vi "User Plugin.vi"(5 "Initialize":bool, 8 "error in (no error)":errorcluster, 10 "ParamValues":sgl[](array[numeric]), 11 "DSI Reference":refnum<class "DCM-DSI-UserFuelExample.lvclass">) -> (0 "error out":errorcluster, 3 "DSI Reference":refnum<class "DCM-DSI-UserFuelExample.lvclass">, 4 "Results":T1[](array[typedef]), 6 "ParamNames":string[](array[string]))   [LabVIEW 2016, in "DCM-DSI-UserFuelExample.lvclass"]
uses:
  DCM-DSI-UserFuelExample.lvclass
  D:/PCG/Products/DCM/Software/DCM-DSI/Classes/DCM-DSI/DCM-DSI.lvclass
  DCM-DSI/UserParameter.ctl
  DCM-DSI/Channel.ctl
  DCM-DSI/Read Channels.vi
  DCM-DSI/Read EPTx Data.vi
  DCM-DSI/Read dt.vi
  DCM-DSI/Write Channels.vi
  DCM-DSI/DCM-DSI.lvclass
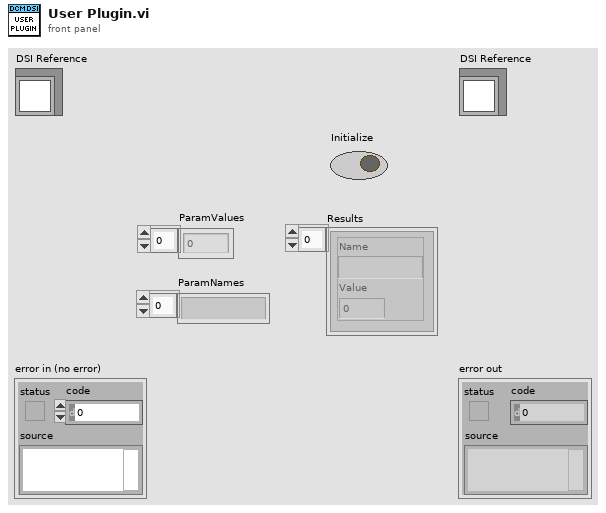
[diagram p1: front panel]
types:
  T1 = typedef "DCM-DSI.lvclass/UserParameter.ctl" = cluster{"Name":string, "Value":dbl}
  T2 = typedef "DCM-DSI.lvclass/Channel.ctl" = cluster{"Name":string, "Unit":string, "Value":sgl}
  T3 = cluster{"XArray":sgl[], "YArray":sgl[], "ZArray":dbl[][]}
  T4 = typedef "EPTx - RevA - RT.lvlib/EPTxData.ctl" = cluster{"Sync":bool, "CurrentCAD":sgl, "Speed [RPM]":sgl, "Config":bool, "Rcvg Primary":bool, "Stall":bool, "Overflow":bool, "Ratio Error":bool, "Pattern Error":bool, "Aux Warning":bool, "Watchdog Error":bool}
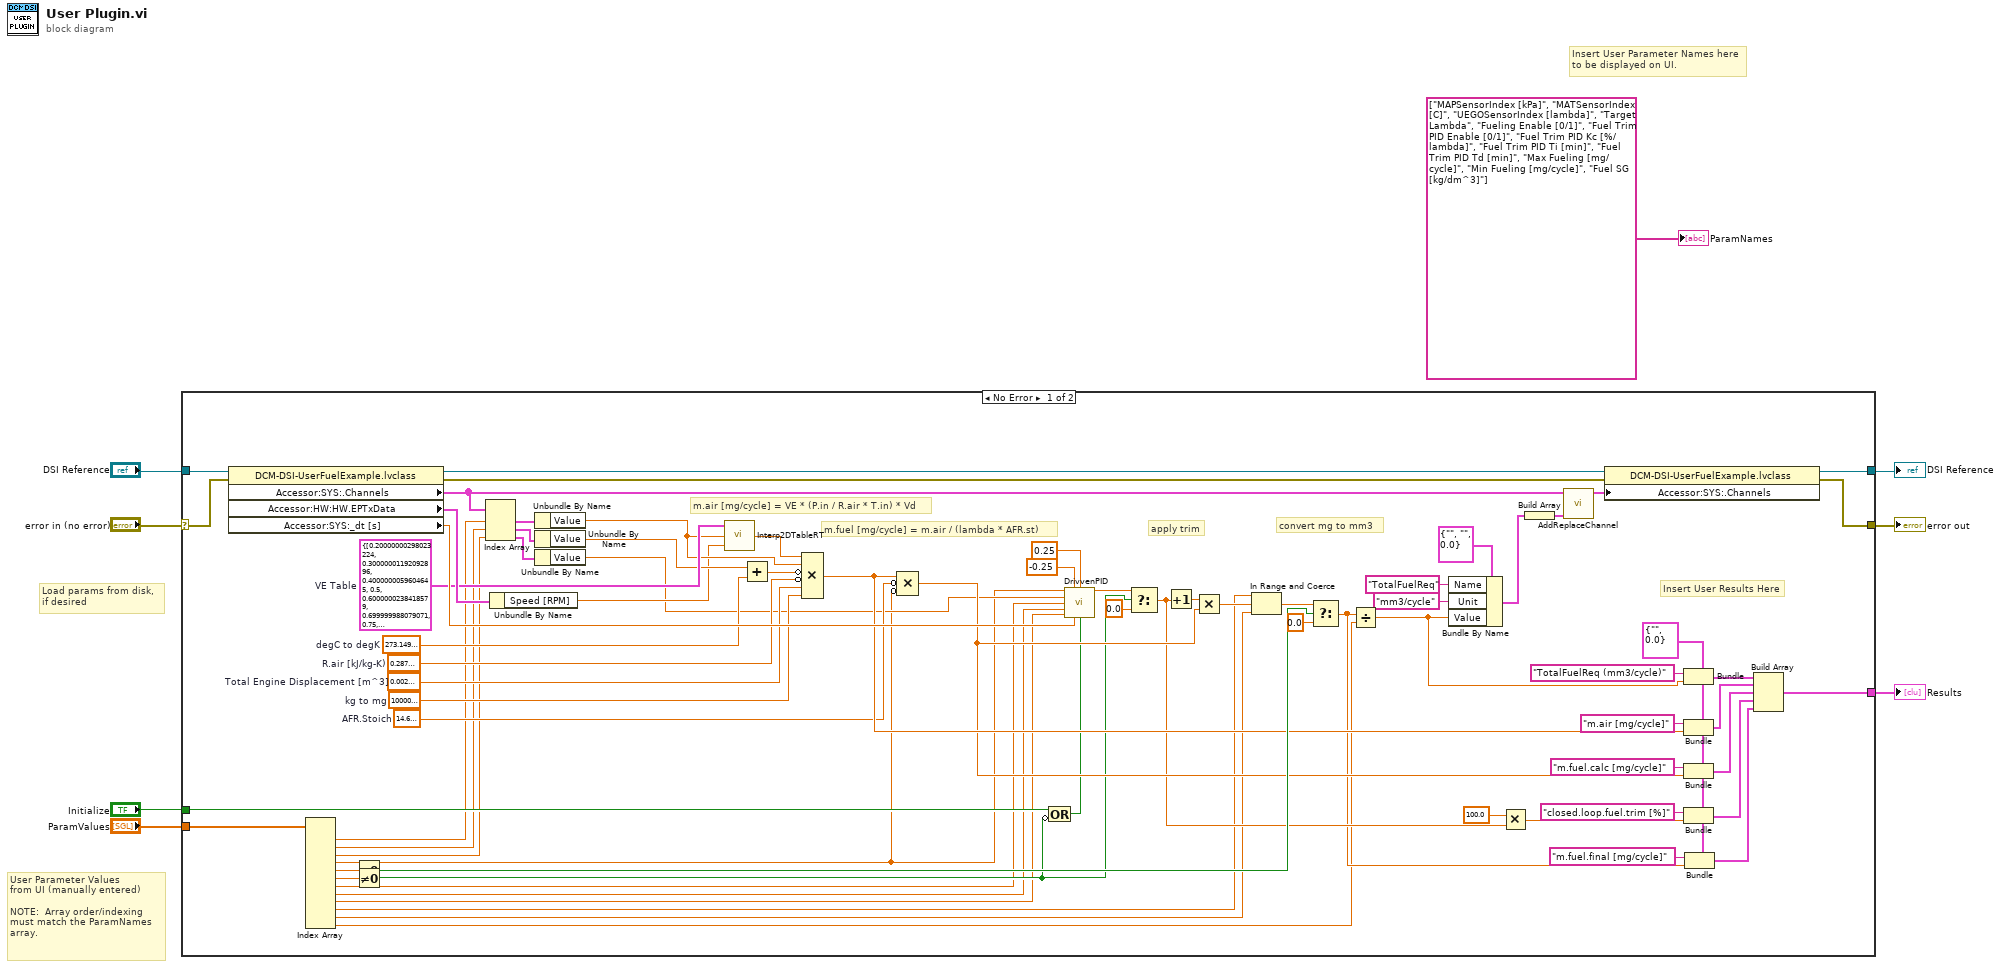
[diagram p0: block diagram]
diagram:
  # "Load params from disk,\nif desired"
  # "User Parameter Values\nfrom UI (manually entered)\n\nNOTE:  Array order/indexing\nmust match the ParamNames\narray."
  # "Insert User Parameter Names here\nto be displayed on UI."
  n1 = case shown="No Error" "error in (no error)" {
    selector: "error in (no error)" -> [w82 w84]
    tunnel: [w81 w84] -> w7
    tunnel: [w79 w83] -> w5
    tunnel: "DSI Reference" -> [w80 w83]
    tunnel: "Initialize" -> [w25 _]
    tunnel: "ParamValues" -> [w78 _]
    tunnel: [w77 _] -> w2
    frame No Error {
      w40 = sgl 1000000.0  # kg to mg
      w41 = sgl 14.7  # AFR.Stoich
      w47 = sgl 0.002  # Total Engine Displacement [m^3]
      w48 = sgl 273.15  # degC to degK
      w51 = sgl 0.287  # R.air [kJ/kg-K)
      w54 = T3 {"XArray"=[0.2, 0.3, 0.4, 0.5, 0.6, 0.7, 0.75, 0.8, 0.85, 0.9, 0.95], "YArray"=[500.0, 1000.0, 1500.0, 2000.0, 2500.0, 3000.0, 3500.0, 4000.0, 4500.0, 5000.0, 5500.0], "ZArray"=[[0.7, 0.7, 0.7, 0.7, 0.7, 0.7, 0.7, 0.7, 0.7, 0.7, 0.7], [0.7, 0.7, 0.7, 0.7, 0.7, 0.7, 0.7, 0.7, 0.7, 0.7, 0.7], [0.7, 0.7, 0.7, 0.7, 0.7, 0.7, 0.7, 0.7, 0.7, 0.7, 0.7], [0.7, 0.7, 0.7, 0.7, 0.7, 0.7, 0.7, 0.7, 0.7, 0.7, 0.7], [0.7, 0.7, 0.7, 0.7, 0.7, 0.7, 0.7, 0.7, 0.7, 0.7, 0.7], [0.7, 0.7, 0.7, 0.7, 0.7, 0.7, 0.7, 0.7, 0.7, 0.7, 0.7], [0.7, 0.7, 0.7, 0.7, 0.7, 0.7, 0.7, 0.7, 0.7, 0.7, 0.7], [0.7, 0.7, 0.7, 0.7, 0.7, 0.7, 0.7, 0.7, 0.7, 0.7, 0.7], [0.7, 0.7, 0.7, 0.7, 0.7, 0.7, 0.7, 0.7, 0.7, 0.7, 0.7], [0.7, 0.7, 0.7, 0.7, 0.7, 0.7, 0.7, 0.7, 0.7, 0.7, 0.7], [0.7, 0.7, 0.7, 0.7, 0.7, 0.7, 0.7, 0.7, 0.7, 0.7, 0.7]]}  # VE Table
      w38 = T1 {"Name"="", "Value"=0.0} ("User Parameter")
      # "apply trim"
      # "convert mg to mm3"
      # "m.fuel [mg/cycle] = m.air / (lambda * AFR.st)"
      # "m.air [mg/cycle] = VE * (P.in / R.air * T.in) * Vd"
      # "Insert User Results Here"
      n2 = property class="DCM-DSI-UserFuelExample.lvclass"(reference=w80, error in=w82) -> (reference out=w73:refnum<class "DCM-DSI-UserFuelExample.lvclass">, error out=w74:errorcluster, "Accessor:SYS:.Channels"=w66:T2[], "Accessor:HW:HW.EPTxData"=w55:T4, "Accessor:SYS:_dt [s]"=w71:sgl)
      n3 = Index Array(array=w78) -> (element #1=w14:sgl, element #2=w13:sgl, element #3=w12:sgl, element #4=w10:sgl, element #5=w9:sgl, element #6=w18:sgl, element #7=w17:sgl, element #8=w16:sgl, element #9=w15:sgl, element #10=w22:sgl, element #11=w21:sgl, element #12=w11:sgl)  [unwired: 12 in]
      n4 = Not Equal To 0?(x=w9) -> (x != 0?=w68:bool)
      n5 = Not Equal To 0?(x=w18) -> (x != 0?=w23:bool)
      n6 = Index Array(array=w66, index #1=w14, index #2=w13, index #3=w12) -> (element #1=w72:T2, element #2=w52:T2, element #3=w42:T2)
      n7 = Unbundle By Name(w55) -> ("Speed [RPM]"=w44:sgl)
      n8 = Unbundle By Name(w72) -> ("Value"=w45:sgl)
      n9 = Unbundle By Name(w52) -> ("Value"=w49:sgl)
      n10 = Unbundle By Name(w42) -> ("Value"=w26:sgl)
      n11 = call <vilib>:"Interp2DTableRT.vi"("Y"=w44, "X"=w45, "2DTable"=w54) -> ("Z"=w46:sgl)
      n12 = Add(x=w49, y=w48) -> (x+y=w50:sgl)
      n13 = Compound Arithmetic op=MULTIPLY(w46, w45, invert w50, invert w51, w47, w40) -> (w43:sgl)
      n14 = Compound Arithmetic op=MULTIPLY(w43, invert w41, invert w10) -> (w34:sgl)
      n15 = Compound Arithmetic op=OR(w25, invert w23) -> (w24:bool)
      n16 = call <vilib>:"DrivvenPID.vi"("Setpoint"=w10, "OutputLow"=sgl -0.25, "OutputHigh"=sgl 0.25, "ProcessVariable"=w26, "ProportionalGain (Kc)"=w17, "IntegralTime (Ti, min)"=w16, "DerivativeTime (Td, min)"=w15, "dt (s)"=w71, "Reinitialize? (F)"=w24) -> ("Output"=w53:sgl)  [unwired: 1 in, 5 out]
      n17 = Select(t=w53, s=w23, f=sgl 0.0) -> (s? t:f=w33:sgl)
      n18 = Increment(x=w33) -> (x+1=w29:sgl)
      n19 = Multiply(x=w29, y=w34) -> (x*y=w32:sgl)
      n20 = In Range and Coerce(upper limit=w22, x=w32, lower limit=w21) -> (coerced(x)=w67:sgl)  [unwired: 1 out]
      n21 = Select(t=w67, s=w68, f=sgl 0.0) -> (s? t:f=w19:sgl)
      n22 = Divide(x=w19, y=w11) -> (x/y=w20:sgl)
      n23 = Bundle By Name(cluster=T2 {"Name"="", "Unit"="", "Value"=0.0} ("Channel In"), "Name"="TotalFuelReq", "Unit"="mm3/cycle", "Value"=w20) -> (w62:T2)
      n24 = Multiply(x=sgl 100.0, y=w33) -> (x*y=w27:sgl)
      n25 = Build Array(w62) -> (w61:T2[])
      n26 = call "AddReplaceChannel.vi"("Channel In"=w61, "Channels in"=w66) -> ("Channels out"=w65:T2[])  [unwired: 9 in]
      n27 = property class="DCM-DSI-UserFuelExample.lvclass"(reference=w73, error in=w74, "Accessor:SYS:.Channels"=w65) -> (reference out=w79:refnum<class "DCM-DSI-UserFuelExample.lvclass">, error out=w81:errorcluster)
      n28 = Bundle(cluster=w38, "Name"="TotalFuelReq (mm3/cycle)", "Value"=w20) -> (w75:T1)
      n29 = Bundle(cluster=w38, "Name"="m.air [mg/cycle]", "Value"=w43) -> (w59:T1)
      n30 = Bundle(cluster=w38, "Name"="m.fuel.calc [mg/cycle]", "Value"=w34) -> (w58:T1)
      n31 = Bundle(cluster=w38, "Name"="closed.loop.fuel.trim [%]", "Value"=w27) -> (w36:T1)
      n32 = Bundle(cluster=w38, "Name"="m.fuel.final [mg/cycle]", "Value"=w19) -> (w35:T1)
      n33 = Build Array(w75, w59, w58, w36, w35) -> (w77:T1[])
    }
    frame Error {
    }
  }
  "error out" <- w7
  "DSI Reference" <- w5
  "Results" <- w2
  "ParamNames" <- string[] ["MAPSensorIndex [kPa]", "MATSensorIndex [C]", "UEGOSensorIndex [lambda]", "Target Lambda", "Fueling Enable [0/1]", "Fuel Trim PID Enable [0/1]", "Fuel Trim PID Kc [%/lambda]", "Fuel Trim PID Ti [min]", "Fuel Trim PID Td [min]", "Max Fueling [mg/cycle]", "Min Fueling [mg/cycle]", "Fuel SG [kg/dm^3]"] ("ParamNames")
